vi "CSM - Reset to Default.vi"(8 "error in (no error)":errorcluster) -> (2 "error out":errorcluster)   [LabVIEW 2017, in "INI-Static-Variable-Support.lvlib"]
doc: "Resets the configuration to default values. All variables will be cleared, and all configurations will be reloaded from the currently loaded configuration files.\n\n\n> [!NOTE] <b>CSM INI-Variable Configuration File Path</b>\n>\n> - <b>Development State</b>: The first INI configuration file found in the Application Directory. If no configuration file exists, it defaults to `csm-app.ini`.\n> - <b>Post-Compilation</b>: An INI configuration file in the same directory as the executable file, with the same name as the executable. LabVIEW automatically generates this file after compilation.\n> - Supports loading multiple configuration files. Configuration items in files loaded later will overwrite identical items in previously loaded files.\n> - Configuration files can use the `[__include]` section to reference other configuration files.\n> - Supports both relative and absolute paths.\n> - Relative paths are relative to the path of the current configuration file.\n> - The name of the configuration file in the `[__include]` section is not critical, as long as the path is correct.\n> - To avoid circular references, the same configuration file will be automatically ignored if loaded a second time."
uses:
  INI-Static-Variable-Support.lvlib
  _Support/_fgv-oper.ctl
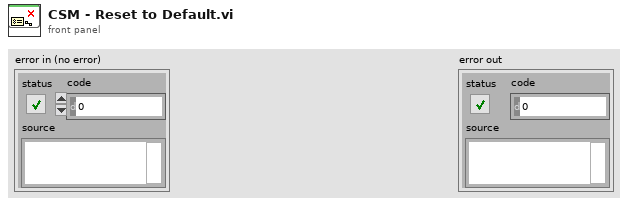
[diagram p1: front panel]
types:
  T1 = typedef "INI-Static-Variable-Support.lvlib/_fgv-oper.ctl" = enum16{"Read", "Write", "Sync", "Sessions", "List Keys", "Load", "List Files", "List Variables", "List Permanent Variables", "Mark Temp Variable as Permenent", "unload", "INIConfig(Memory)", "Reset", "Restore Variable Value"}
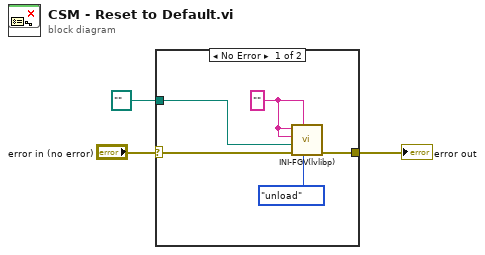
[diagram p0: block diagram]
diagram:
  n1 = case shown="No Error" "error in (no error)" {
    selector: "error in (no error)" -> [w6 w9]
    tunnel: path "" ("Path") -> [w7 _]
    tunnel: [w5 w9] -> w1
    frame No Error {
      w4 = "" (">> Variable Name >>")
      n2 = call "INI-FGV(lvlibp).vi"("Enum"=_fgv-oper."unload", "Prefered Section"=w4, "error IN"=w6, "Path"=w7, ">> Default Value >>"=w4, ">> Variable Name >>"=w4) -> ("error out"=w5:errorcluster)  [unwired: 2 in, 3 out]
    }
    frame Error {
    }
  }
  "error out" <- w1
